vi "7-29-19 Increasing.vi"() -> ()   [LabVIEW 2020]
uses:
  <vilib>/Analysis/NI_AALPro.lvlib
  <vilib>/Analysis/NI_AALBase.lvlib
  <vilib>/Analysis/baseanly.llb/Mean (DBL).vi
  <userlib>/LevyLab/LV to ITX/Data/Data.lvclass
panel:
  out "G vs Temp":cluster{"Data":dbl[], "Data":dbl[]}[](graph)
  out "G vs Time":cluster{"Data":dbl[], "Data":dbl[]}[](graph)
  out "dG/dt/G vs temp":cluster{"Data":dbl[], "Data":dbl[]}[](graph)
  out "dG/dt Vs Temp Normalized":cluster{"Data":dbl[], "Data":dbl[]}[](graph)
  out "Slopes":cluster{dbl[], dbl[]}
  out "G Vs Time Fitted":cluster{"Data":dbl[], "Data":dbl[]}[](graph)
  out "G Vs Time":cluster{"Data":dbl[], "Data":dbl[]}[](graph)
  out "Data":dbl[][](array[numeric])
  in  "File Path":path=path "G:/My Drive/Data/7-30 Increasing SA03083.dat"
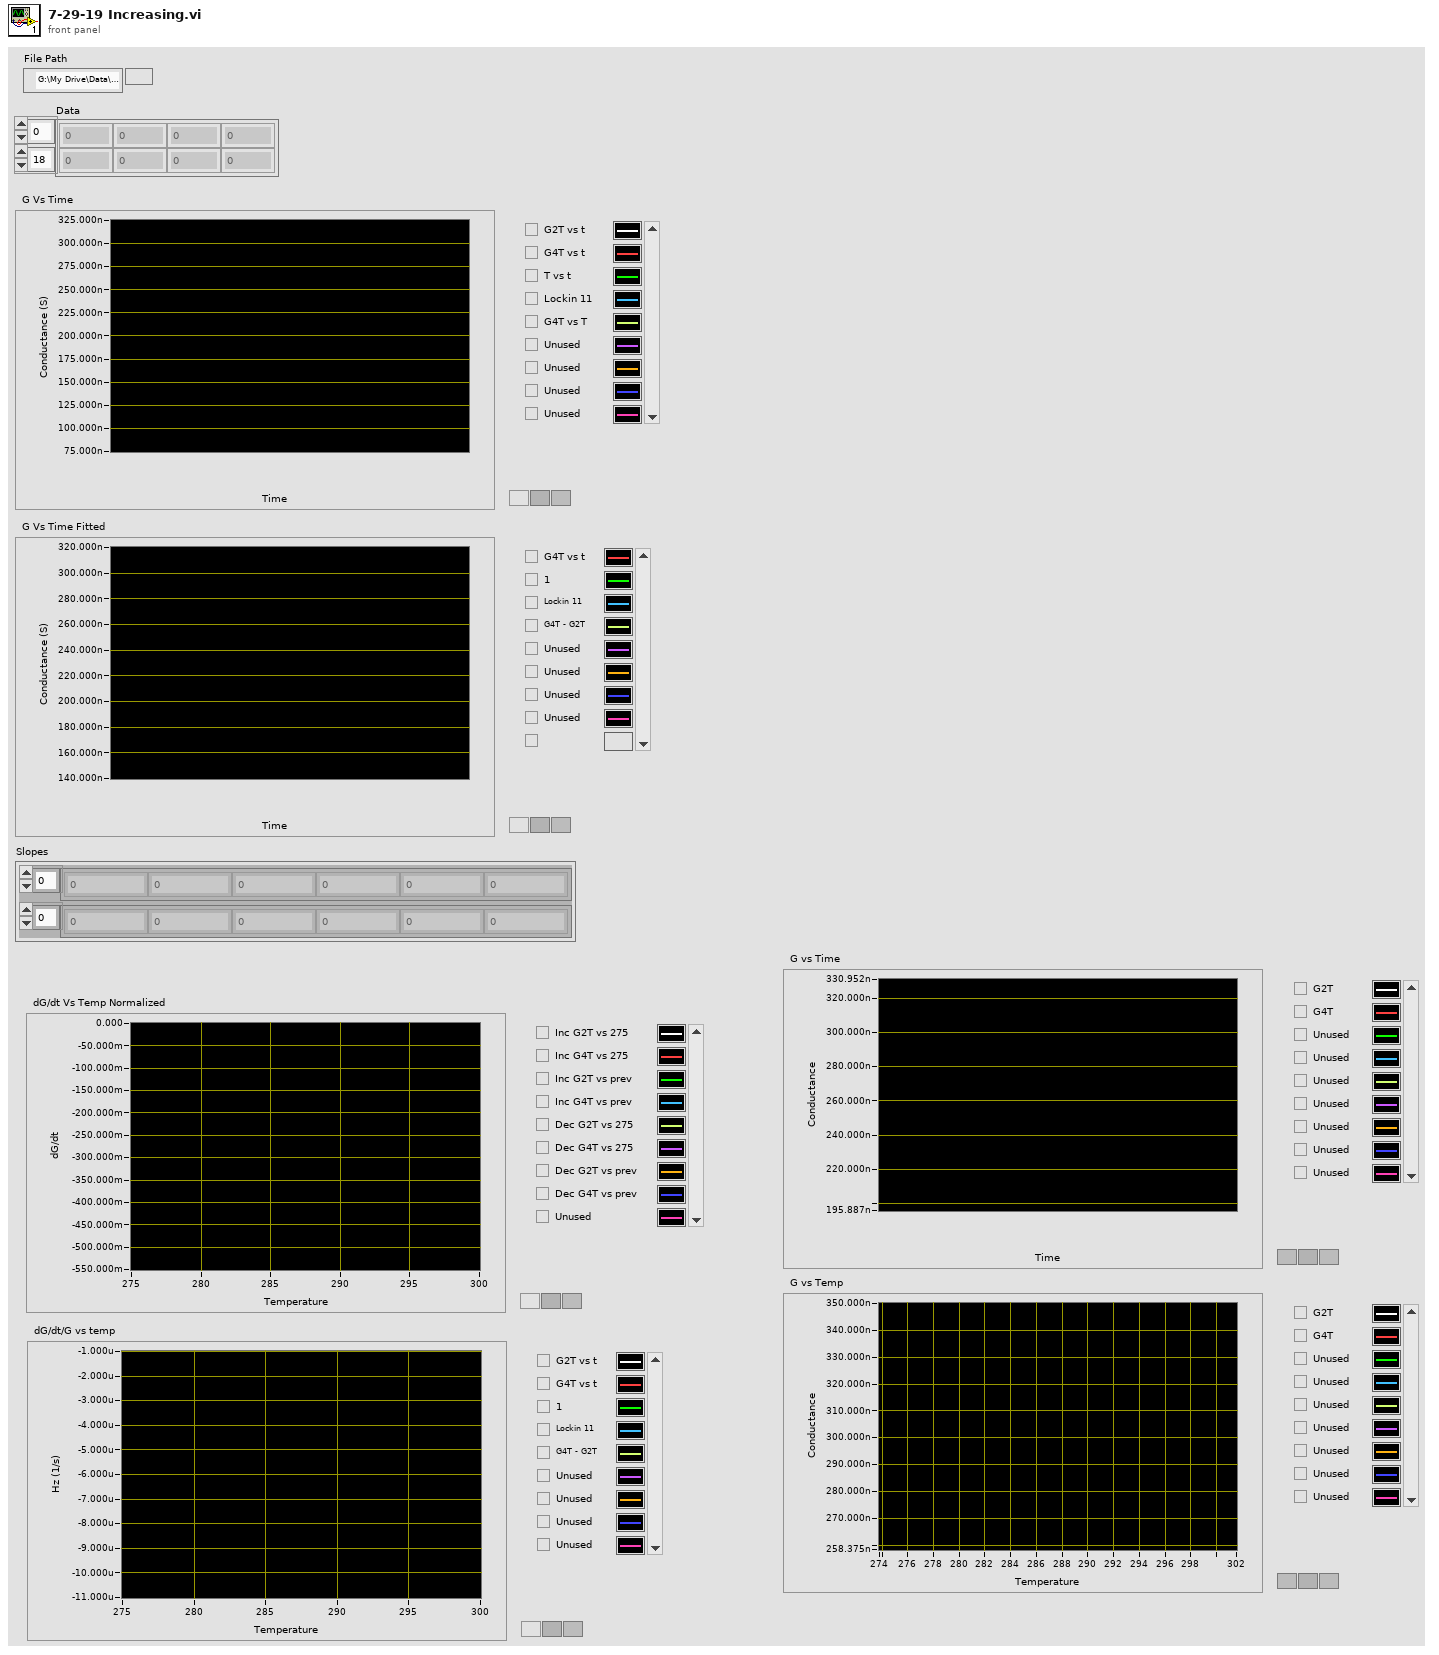
[diagram p1: front panel]
types:
  T1 = typedef "Data.lvclass/Dictionary--cluster.ctl" = cluster{"key":string, "value":variant}
  T2 = cluster{"Data (Dictionary)":T1[], cluster{"key":dbl, "value":dbl}[]}
  T3 = cluster{"Data (Dictionary)":T1[], "Data (Dictionary)":T1[]}
  T4 = cluster{"slope min":dbl, "slope max":dbl, "intercept min":dbl, "intercept max":dbl}
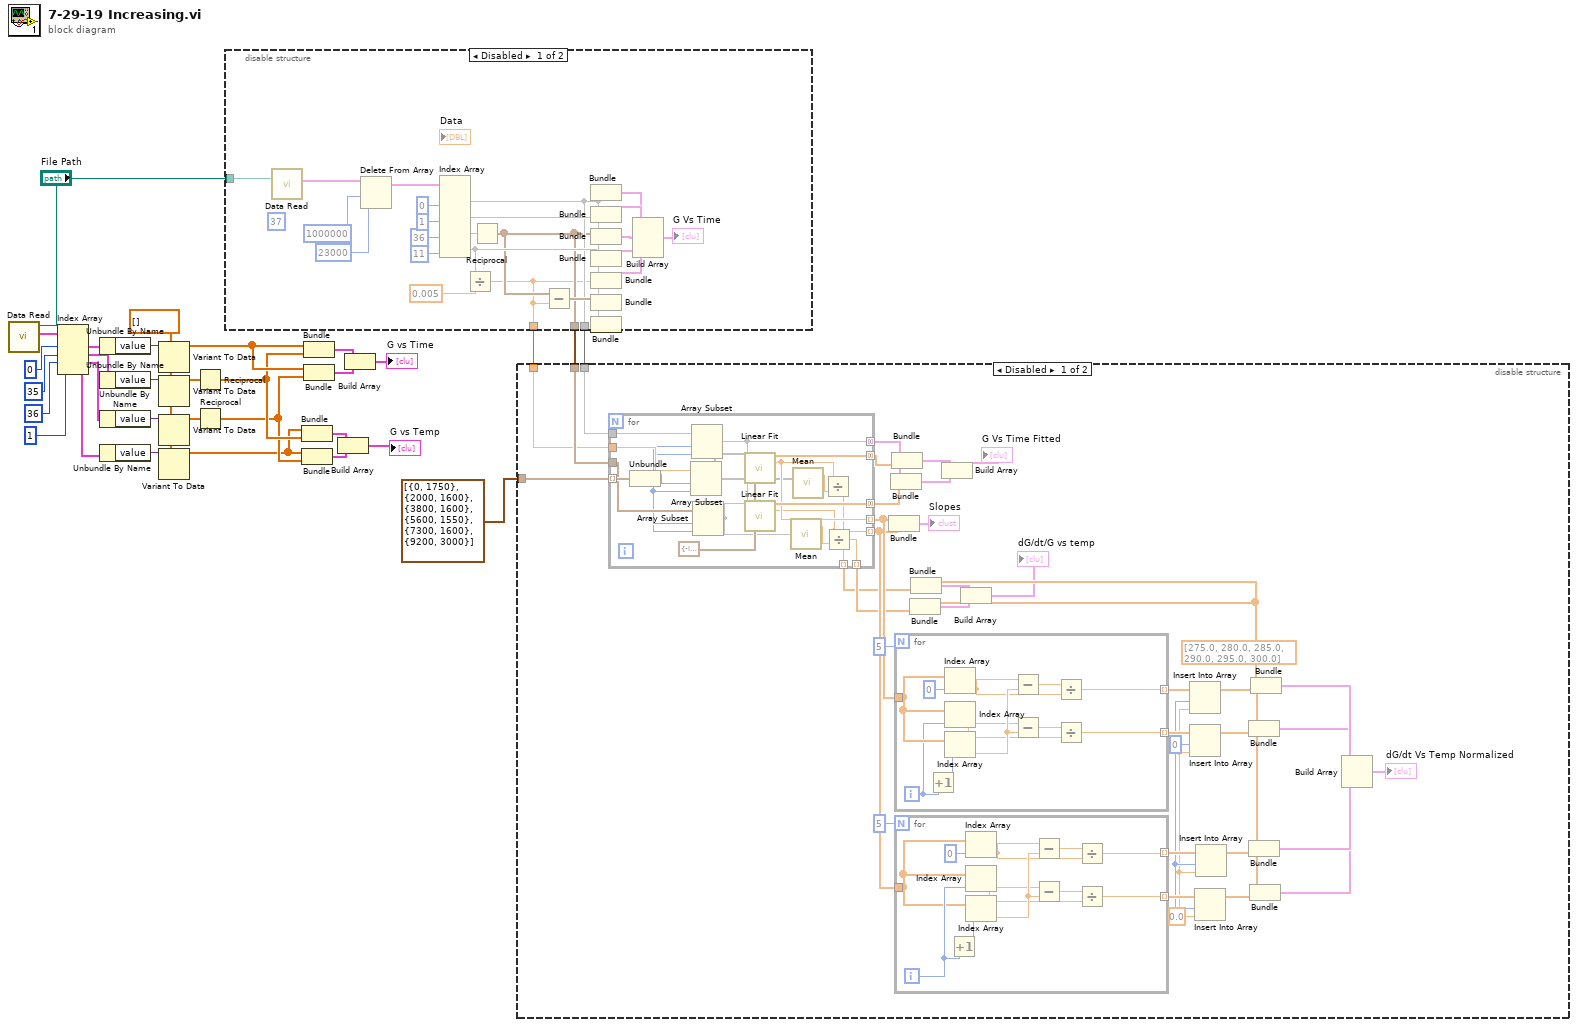
[diagram p0: block diagram]
diagram:
  w22 = dbl[] []
  n1 = call <userlib>:"Data Read.vi"("path"="File Path") -> ("Data (Dictionary)"=w23:T1[])  [unwired: 7 in, 3 out]
  n2 = Index Array(array=w23, index #1=0 ("disabled index (col)"), index #2=35 ("index (col)"), index #3=36 ("index (col)"), index #4=1 ("index (col)")) -> (element #1=w17:T1, element #2=w16:T1, element #3=w15:T1, element #4=w14:T1)
  n3 = Unbundle By Name(w17) -> ("value"=w27:variant)
  n4 = Unbundle By Name(w16) -> ("value"=w26:variant)
  n5 = Unbundle By Name(w15) -> ("value"=w24:variant)
  n6 = Unbundle By Name(w14) -> ("value"=w25:variant)
  n7 = Variant To Data(type=w22, Variant=w27) -> (data=w11:dbl[])  [unwired: 1 in, 1 out]
  n8 = Variant To Data(type=w22, Variant=w26) -> (data=w12:dbl[])  [unwired: 1 in, 1 out]
  n9 = Variant To Data(type=w22, Variant=w24) -> (data=w13:dbl[])  [unwired: 1 in, 1 out]
  n10 = Variant To Data(type=w22, Variant=w25) -> (data=w8:dbl[])  [unwired: 1 in, 1 out]
  n11 = Reciprocal(x=w12) -> (1/x=w10:dbl[])
  n12 = Reciprocal(x=w13) -> (1/x=w9:dbl[])
  n13 = disable-structure shown="Disabled" {
    disable-tunnel: [w36 _] -> w30
    disable-tunnel: [w35 _] -> w29
    disable-tunnel: [w34 _] -> w28
    disable-tunnel: "File Path" -> [w32 _]
    frame Disabled {
      (unwired) 37 ("header length")
      n14 = call <userlib>:"Data Read.vi"("path"=w32) -> ("Data (Dictionary)"=w33:T1[])  [unwired: 7 in, 3 out]
      n15 = Delete From Array(array=w33, length=1000000, index=23000) -> (array with subset deleted=w37:T1[])  [unwired: 1 out]
      n16 = Index Array(array=w37, index (col) #1=0 ("disabled index (col)"), index (col) #2=1 ("index (col)"), index (col) #3=36 ("index (col)"), index (col) #4=11 ("index (col)")) -> (element #1=w36:T1[], element #2=w52:T1[], element #3=w45:T1[], element #4=w38:T1[])  [unwired: 4 in]
      n17 = Divide(x=w38, y=0.005) -> (x/y=w34:dbl)
      n18 = Reciprocal(x=w45) -> (1/x=w35:cluster{"key":dbl, "value":dbl}[])
      n19 = Subtract(x=w35, y=w34) -> (x-y=w41:cluster{"key":dbl, "value":dbl}[])
      n20 = Bundle("Data (Dictionary)"=w36, w34) -> (w44:cluster{"Data (Dictionary)":T1[], dbl})  [unwired: 1 in]
      n21 = Bundle("Data (Dictionary)"=w36, w35) -> (w51:T2)  [unwired: 1 in]
      n22 = Bundle("Data (Dictionary)"=w36, "Data (Dictionary)"=w52) -> (w50:T3)  [unwired: 1 in]
      n23 = Bundle("Data (Dictionary)"=w36, "Data (Dictionary)"=w38) -> (w49:T3)  [unwired: 1 in]
      n24 = Bundle("Data (Dictionary)"=w36, w41) -> (w42:T2)  [unwired: 1 in]
      n25 = Bundle("Data (Dictionary)"=w52, w34) -> ()  [unwired: 1 in, 1 out]
      n26 = Bundle("Data (Dictionary)"=w52, w35) -> ()  [unwired: 1 in, 1 out]
      n27 = Build Array(w44, w51, w50, w49, w42) -> (→"G Vs Time":cluster{"Data (Dictionary)":T1[], dbl}[])
    }
    frame Enabled {
    }
  }
  n28 = Bundle(w8, w10) -> (w3:cluster{dbl[], dbl[]})  [unwired: 1 in]
  n29 = Bundle(w8, w9) -> (w4:cluster{dbl[], dbl[]})  [unwired: 1 in]
  n30 = Bundle(w11, w10) -> (w6:cluster{dbl[], dbl[]})  [unwired: 1 in]
  n31 = Bundle(w11, w9) -> (w7:cluster{dbl[], dbl[]})  [unwired: 1 in]
  n32 = Build Array(w3, w4) -> (→"G vs Temp":cluster{dbl[], dbl[]}[])
  n33 = Build Array(w6, w7) -> (→"G vs Time":cluster{dbl[], dbl[]}[])
  n34 = disable-structure shown="Disabled" {
    disable-tunnel: cluster{"Index":i32, "Length":i32}[] [{"Index"=0, "Length"=1750}, {"Index"=2000, "Length"=1600}, {"Index"=3800, "Length"=1600}, {"Index"=5600, "Length"=1550}, {"Index"=7300, "Length"=1600}, {"Index"=9200, "Length"=3000}] -> [w90 _]
    disable-tunnel: w30 -> [w82 _]
    disable-tunnel: w29 -> [w57 _]
    disable-tunnel: w28 -> [w56 _]
    frame Disabled {
      w58 = dbl[] [275.0, 280.0, 285.0, 290.0, 295.0, 300.0]
      w75 = 0.0 ("new element/subarray")
      w76 = 0 ("index")
      n35 = for {
        tunnel: w90 -> [w130] mode=indexing
        tunnel: w56 -> [w129]
        tunnel: w57 -> [w128]
        tunnel: [w124] -> w87 mode=concatenating
        tunnel: [w123] -> w86 mode=concatenating
        tunnel: [w118] -> w65 mode=indexing
        tunnel: [w117] -> w64 mode=indexing
        tunnel: [w122] -> w88 mode=concatenating
        tunnel: w82 -> [w121]
        tunnel: [w116] -> w59 mode=indexing
        tunnel: [w115] -> w60 mode=indexing
        w125 = T4 {"slope min"=-inf, "slope max"=inf, "intercept min"=-inf, "intercept max"=inf} ("parameter bounds")
        n36 = Unbundle(w130) -> ("Index"=w127:i32, "Length"=w126:i32)
        n37 = Array Subset(array=w129, index=w127, length=w126) -> (w114:void[])
        n38 = Array Subset(array=w121, index=w127, length=w126) -> (w122:T1[])
        n39 = Array Subset(array=w128, index=w127, length=w126) -> (w113:cluster{"key":dbl, "value":dbl}[])
        n40 = call <vilib>:"Linear Fit.vi"("Y"=w114, "X"=w122, "parameter bounds"=w125) -> ("Best Linear Fit"=w124:dbl[], "slope"=w118:dbl)  [unwired: 8 in, 3 out]
        n41 = call <vilib>:"Linear Fit.vi"("Y"=w113, "X"=w122, "parameter bounds"=w125) -> ("Best Linear Fit"=w123:dbl[], "slope"=w117:dbl)  [unwired: 8 in, 3 out]
        n42 = call-poly <vilib>:"Mean.vi"("X"=w113) -> ("mean"=w120:dbl)  [unwired: 1 out]
        n43 = call-poly <vilib>:"Mean.vi"("X"=w114) -> ("mean"=w119:dbl)  [unwired: 1 out]
        n44 = Divide(x=w118, y=w119) -> (x/y=w116:dbl)
        n45 = Divide(x=w117, y=w120) -> (x/y=w115:dbl)
      }
      n46 = Bundle(w65, w64) -> (→"Slopes":cluster{dbl[], dbl[]})  [unwired: 1 in]
      n47 = Bundle(w88, "Best Linear Fit"=w86) -> (w85:cluster{T1[], "Best Linear Fit":dbl[]})  [unwired: 1 in]
      n48 = Bundle(w88, "Best Linear Fit"=w87) -> (w84:cluster{T1[], "Best Linear Fit":dbl[]})  [unwired: 1 in]
      n49 = for {
        N: 5 -> [_]
        tunnel: w65 -> [w112]
        tunnel: [w105] -> w80 mode=indexing
        tunnel: [w104] -> w79 mode=indexing
        i -> [w110]
        n50 = Increment(x=w110) -> (x+1=w111:i32)
        n51 = Index Array(array=w112, index=0) -> (element=w103:dbl)
        n52 = Index Array(array=w112, index=w110) -> (element=w102:dbl)
        n53 = Index Array(array=w112, index=w111) -> (element=w106:dbl)
        n54 = Subtract(x=w103, y=w106) -> (x-y=w108:dbl)
        n55 = Subtract(x=w102, y=w106) -> (x-y=w107:dbl)
        n56 = Divide(x=w108, y=w103) -> (x/y=w105:dbl)
        n57 = Divide(x=w107, y=w102) -> (x/y=w104:dbl)
      }
      n58 = for {
        N: 5 -> [_]
        tunnel: w64 -> [w95]
        tunnel: [w94] -> w78 mode=indexing
        tunnel: [w93] -> w77 mode=indexing
        i -> [w96]
        n59 = Increment(x=w96) -> (x+1=w97:i32)
        n60 = Index Array(array=w95, index=0) -> (element=w91:dbl)
        n61 = Index Array(array=w95, index=w96) -> (element=w92:dbl)
        n62 = Index Array(array=w95, index=w97) -> (element=w101:dbl)
        n63 = Subtract(x=w91, y=w101) -> (x-y=w99:dbl)
        n64 = Subtract(x=w92, y=w101) -> (x-y=w100:dbl)
        n65 = Divide(x=w99, y=w91) -> (x/y=w94:dbl)
        n66 = Divide(x=w100, y=w92) -> (x/y=w93:dbl)
      }
      n67 = Bundle(w58, w60) -> (w61:cluster{dbl[], dbl[]})  [unwired: 1 in]
      n68 = Bundle(w58, w59) -> (w62:cluster{dbl[], dbl[]})  [unwired: 1 in]
      n69 = Build Array(w84, w85) -> (→"G Vs Time Fitted":cluster{T1[], "Best Linear Fit":dbl[]}[])
      n70 = Build Array(w62, w61) -> (→"dG/dt/G vs temp":cluster{dbl[], dbl[]}[])
      n71 = Insert Into Array(array=w80, index=w76, new element=w75) -> (w72:dbl[])
      n72 = Insert Into Array(array=w79, index=w76, new element=w75) -> (w71:dbl[])
      n73 = Insert Into Array(array=w77, index=w76, new element=w75) -> (w73:dbl[])
      n74 = Insert Into Array(array=w78, index=w76, new element=w75) -> (w74:dbl[])
      n75 = Bundle(w58, w71) -> (w68:cluster{dbl[], dbl[]})  [unwired: 1 in]
      n76 = Bundle(w58, w74) -> (w70:cluster{dbl[], dbl[]})  [unwired: 1 in]
      n77 = Bundle(w58, w73) -> (w67:cluster{dbl[], dbl[]})  [unwired: 1 in]
      n78 = Bundle(w58, w72) -> (w69:cluster{dbl[], dbl[]})  [unwired: 1 in]
      n79 = Build Array(w69, w70, w68, w67) -> (→"dG/dt Vs Temp Normalized":cluster{dbl[], dbl[]}[])
    }
    frame Enabled {
    }
  }
